vi "Curtin1_soundcards.vi"(6 "hush?":bool, 8 "Settings In":T1={"Name of test"="", "Date"=timestamp(0 s since 1904-01-01), "Location"="", "Template"="", "Soundcard"="", "resolution"=32, "Sampling rate"=48000, "Ch1 Gain "=25.0, "Ch2 Gain"=10.0, "Sample time (s)"=0.3, "Pre-trigger (s)"=0.01, "Hammer Threshold"=10.0, "Positions"=12, "Taps/Position"=5, "Set Names"="", "Freq resolution"=10.0, "Hammer cutoff"=0.0, "Mic cutoff"=0.0, "Double bounce "=0.0, "Hammer Cal"=10.0, "dB Offset"=0.0, "Accel Cal"=10.0, "Vibrometer Cal"=0.0, "Mic Cal"=0.0, "Output"=2, "Voltage Cal"=1.0, "Vibrometer Port"="ASRL27::INSTR", "Range"=4, "High Pass"=2, "Bandwidth"=4, "X Range"=[], "Y Range"=[], "dB Spread"=0.0, "Trigger"=0, "Ch_1"=25, "Ch_2"=25, "flip?"=FALSE, "60Hz"=FALSE, "Time offset"=0.0, "Piezo Cal"=1.0, "Default Notes"=""} {"Ch_2" min=1 step=1; "Ch_1" min=1 max=100 step=1; "Trigger" items=["Hammer (force)", "Self-tap", "Spacebar"]; "Bandwidth" items=["1 kHz"=1, "5 kHz"=5, "10 kHz"=10, "25 kHz"=25, "50 kHz"=50, "100 kHz"=100]; "High Pass" items=["Off", "13 Hz", "104 Hz"]; "Range" items=["10 mm/s"=1, "20 mm/s"=2, "50 mm/s"=5, "100 mm/s"=10, "200 mm/s"=20, "500 mm/s"=50, "1 m/s"=100, "2 m/s"=200]; "Output" items=["Accelerometer", "Speed (from acceleration)", "Microphone", "Vibrometer", "Piezo"]; "Voltage Cal" format="%#_13g"; "Ch2 Gain" format="%#_13g"; "Ch1 Gain" format="%#_13g"; "Double bounce" min=0.0; "Mic cutoff" min=0.0 format="%#_4g"; "Hammer cutoff" min=0.0 format="%#_4g"; "Freq resolution" min=0.0; "Pre-trigger (s)" format="%#_13g"; "Date" format="%<%H:%M\n%d/%m/%y>T"; "resolution" items=["16 bit"=16, "24 bit"=24, "32 bit"=32]; "Sampling rate" items=["22050 samp/s"=22050, "44100 samp/s"=44100, "48000 samp/s"=48000]}, 11 "device:":refnum<vi>) -> (0 "Settings Out":T1={"Name of test"="", "Date"=timestamp(0 s since 1904-01-01), "Location"="", "Template"="", "Soundcard"="", "resolution"=32, "Sampling rate"=48000, "Ch1 Gain "=25.0, "Ch2 Gain"=10.0, "Sample time (s)"=0.3, "Pre-trigger (s)"=0.01, "Hammer Threshold"=10.0, "Positions"=12, "Taps/Position"=5, "Set Names"="", "Freq resolution"=10.0, "Hammer cutoff"=0.0, "Mic cutoff"=0.0, "Double bounce "=0.0, "Hammer Cal"=10.0, "dB Offset"=0.0, "Accel Cal"=10.0, "Vibrometer Cal"=0.0, "Mic Cal"=0.0, "Output"=2, "Voltage Cal"=1.0, "Vibrometer Port"="ASRL27::INSTR", "Range"=4, "High Pass"=2, "Bandwidth"=4, "X Range"=[], "Y Range"=[], "dB Spread"=0.0, "Trigger"=0, "Ch_1"=25, "Ch_2"=25, "flip?"=FALSE, "60Hz"=FALSE, "Time offset"=0.0, "Piezo Cal"=1.0, "Default Notes"=""} {"Ch_2" min=1 step=1; "Ch_1" min=1 max=100 step=1; "Trigger" items=["Hammer (force)", "Self-tap", "Spacebar"]; "Bandwidth" items=["1 kHz"=1, "5 kHz"=5, "10 kHz"=10, "25 kHz"=25, "50 kHz"=50, "100 kHz"=100]; "High Pass" items=["Off", "13 Hz", "104 Hz"]; "Range" items=["10 mm/s"=1, "20 mm/s"=2, "50 mm/s"=5, "100 mm/s"=10, "200 mm/s"=20, "500 mm/s"=50, "1 m/s"=100, "2 m/s"=200]; "Output" items=["Accelerometer", "Speed (from acceleration)", "Microphone", "Vibrometer", "Piezo"]; "Voltage Cal" format="%#_13g"; "Ch2 Gain" format="%#_13g"; "Ch1 Gain" format="%#_13g"; "Double bounce" min=0.0; "Mic cutoff" min=0.0 format="%#_4g"; "Hammer cutoff" min=0.0 format="%#_4g"; "Freq resolution" min=0.0; "Pre-trigger (s)" format="%#_13g"; "Date" format="%<%H:%M\n%d/%m/%y>T"; "resolution" items=["16 bit"=16, "24 bit"=24, "32 bit"=32]; "Sampling rate" items=["22050 samp/s"=22050, "44100 samp/s"=44100, "48000 samp/s"=48000]}, 3 "Devices":string[](array[string]))   [LabVIEW 2022 SP3]
uses:
  PreferencesControl.ctl
  Mic/Mic_Global.vi
panel:
  # "Hz"
  # "dB"
  # "dB"
  # "sec"
  # "sec"
  # "mV/Pa"
  # "mV/m/s2"
  # "mV/mm/s"
  # "V/N"
  # "sec"
  # "sec"
  # "mV/N"
  # "a.u."
  # "a.u."
  # "sec"
  # "Hz"
  # "dB"
  # "dB"
  # "sec"
  # "sec"
  # "mV/Pa"
  # "mV/m/s2"
  # "mV/mm/s"
  # "V/N"
  # "sec"
  # "sec"
  # "mV/N"
  # "a.u."
  # "a.u."
  # "sec"
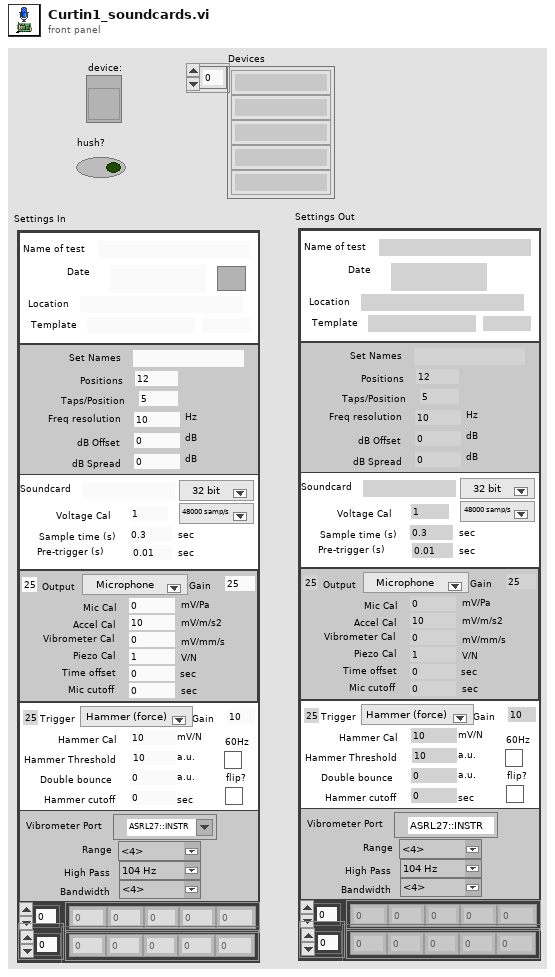
[diagram p1: front panel]
types:
  T1 = typedef "PreferencesControl.ctl" = cluster{"Name of test":string, "Date":timestamp, "Location":string, "Template":string, "Soundcard":string, "resolution":u16, "Sampling rate":u16, "Ch1 Gain ":dbl, "Ch2 Gain":dbl, "Sample time (s)":dbl, "Pre-trigger (s)":dbl, "Hammer Threshold":dbl, "Positions":i16, "Taps/Position":i16, "Set Names":string, "Freq resolution":dbl, "Hammer cutoff":dbl, "Mic cutoff":dbl, "Double bounce ":dbl, "Hammer Cal":dbl, "dB Offset":dbl, "Accel Cal":dbl, "Vibrometer Cal":dbl, "Mic Cal":dbl, "Output":u16, "Voltage Cal":dbl, "Vibrometer Port":refnum<visa-resource-name>, "Range":u16, "High Pass":u16, "Bandwidth":u16, "X Range":cluster{"Minimum":dbl, "Maximum":dbl, "Increment":dbl, "Minor Increment":dbl, "Start":dbl}[], "Y Range":cluster{"Minimum":dbl, "Maximum":dbl, "Increment":dbl, "Minor Increment":dbl, "Start":dbl}[], "dB Spread":dbl, "Trigger":u16, "Ch_1":u8, "Ch_2":u8, "flip?":bool, "60Hz":bool, "Time offset":dbl, "Piezo Cal":dbl, "Default Notes":string}
  T2 = cluster{"channels":i32[], "depths":i32[], "minFreq":dbl, "maxFreq":dbl}
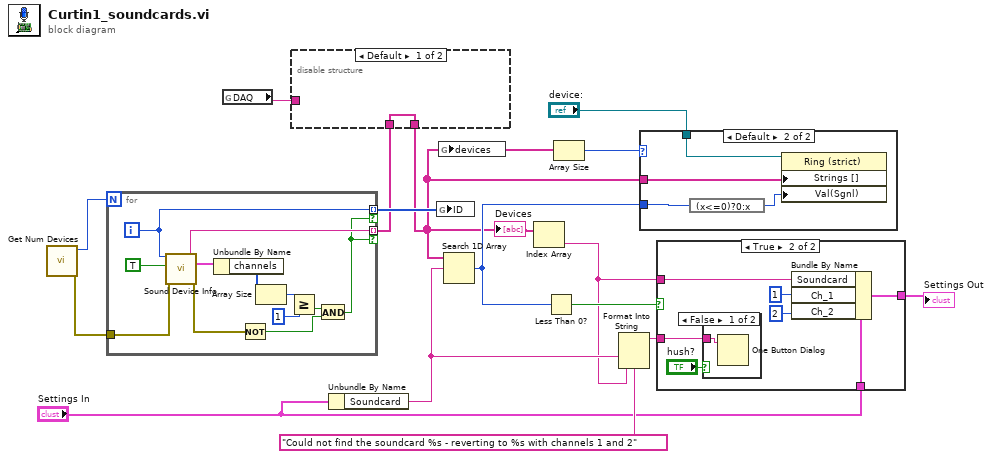
[diagram p0: block diagram]
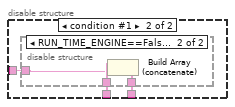
[diagram p2: hidden frame]
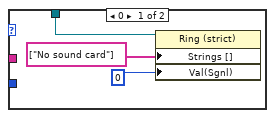
[diagram p4: hidden frame]
diagram:
  n1 = call <vilib>:"Get Num Devices.vi"() -> ("error out"=w15:errorcluster, "Number of Input Devices"=w16:i32)  [unwired: 1 in, 9 out]
  n2 = for {
    N: w16 -> [_]
    tunnel: w15 -> [w27]
    tunnel: [w26] -> w3 mode=indexing if=w17
    tunnel: [w18] -> w7 mode=indexing if=w17
    i -> [w18]
    n3 = call <vilib>:"Sound Device Info.vi"("device"=w18, "isInput?"=TRUE, "error in (no error)"=w27) -> ("Device Name"=w26:string, "Capabilities"=w25:T2, "error out"=w21:errorcluster)  [unwired: 10 out]
    n4 = Unbundle By Name(w25) -> ("channels"=w24:i32[])
    n5 = Not(x=w21) -> (.not. x?=w19:bool)
    n6 = Array Size(array=w24) -> (size(s)=w23:i32)
    n7 = Greater Or Equal?(x=w23, y=1) -> (x >= y?=w20:bool)
    n8 = And(x=w20, y=w19) -> (x .and. y?=w17:bool)
  }
  n9 = global read "Mic_Global.vi" "DAQ"() -> (w1:string)
  n10 = disable-structure shown="Default" {
    disable-tunnel: w3 -> [w29 w32]
    disable-tunnel: [w29 w31] -> w2
    disable-tunnel: w1 -> [_ w30]
    frame condition #0 (active) {
    }
    frame condition #1 {
      n11 = disable-structure shown="RUN_TIME_ENGINE==False" {
        disable-tunnel: w32 -> [w33 w35]
        disable-tunnel: [w33 w36] -> w31
        disable-tunnel: w30 -> [_ w34]
        frame condition #0 {
        }
        frame condition #1 (active) {
          n12 = Build Array (concatenate)(w35, w34) -> (w36:string[])
        }
      }
    }
  }
  "Devices" <- w2
  n13 = Unbundle By Name("Settings In") -> ("Soundcard"=w12:string)
  n14 = global write "Mic_Global.vi" "ID"(w7) -> ()
  n15 = global write "Mic_Global.vi" "devices"(w2) -> ()
  n16 = Search 1D Array(1D array=w2, element=w12) -> (index of element=w9:i32)  [unwired: 1 in]
  n17 = Index Array(array=w2) -> (element=w5:string)  [unwired: 1 in]
  n18 = Less Than 0?(x=w9) -> (x < 0?=w14:bool)
  n19 = Array Size(array=w2) -> (size(s)=w10:i32)
  n20 = Format Into String(format string="Could not find the soundcard %s - reverting to %s with channels 1 and 2" ("message"), w12, w5) -> (resulting string=w11:string)  [unwired: 2 in, 1 out]
  n21 = case shown="Default" w10 {
    tunnel: w2 -> [_ w43]
    tunnel: w9 -> [_ w41]
    tunnel: "device:" -> [w37 w40]
    frame 0 {
      n22 = property on="Property Node" class="Ring (strict)"(reference=w37, "Strings []"=string[] ["No sound card"], "Val(Sgnl)"=0) -> ()  [unwired: 1 in, 2 out]
    }
    frame Default {
      n23 = expression code="(x<=0)?0:x"(w41) -> (w42:i32)
      n24 = property on="Property Node" class="Ring (strict)"(reference=w40, "Strings []"=w43, "Val(Sgnl)"=w42) -> ()  [unwired: 1 in, 2 out]
    }
  }
  n25 = case shown="True" w14 {
    tunnel: w11 -> [_ w51]
    tunnel: "Settings In" -> [w44 w50]
    tunnel: w5 -> [_ w49]
    tunnel: [w44 w46] -> w4
    frame False {
    }
    frame True {
      n26 = case shown="False" "hush?" {
        tunnel: w51 -> [w52 _]
        frame False {
          n27 = One Button Dialog(message=w52) -> ()  [unwired: 1 in, 1 out]
        }
        frame True {
        }
      }
      n28 = Bundle By Name(cluster=w50, "Soundcard"=w49, "Ch_1"=u8 1, "Ch_2"=u8 2) -> (w46:T1)
    }
  }
  "Settings Out" <- w4
